vi "Scope Report Event.vi"(8 "error in (no error)":errorcluster, 9 "Event Data":variant, 10 "Scope Events":T1, 11 "I_Scope in":refnum<class "I_Scope.lvclass">) -> (0 "error out":errorcluster, 3 "I_Scope out":refnum<class "I_Scope.lvclass">)   [LabVIEW 2020, in "Actor_Scope.lvlib" / "I_Scope.lvclass"]
uses:
  I_Scope.lvclass
  Actor_Scope/Scope_Event.ctl
  Actor_Scope/Actor_Scope.lvclass
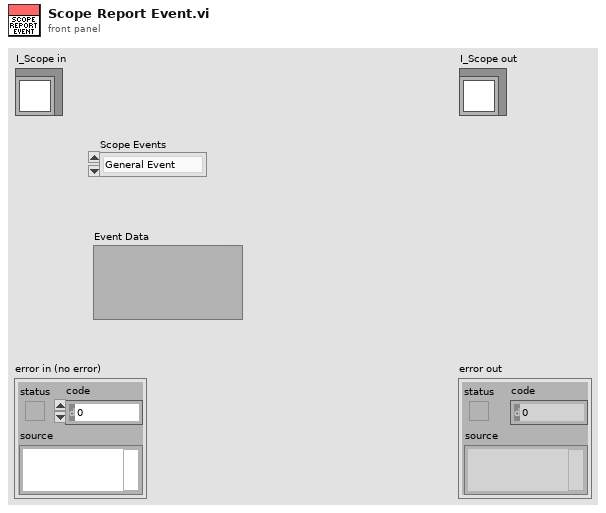
[diagram p1: front panel]
types:
  T1 = typedef "Actor_Scope.lvlib/Actor_Scope.lvclass/Scope_Event.ctl" = enum16{"General Event", "Inited", "Error", "Wfm Acq Complete"}
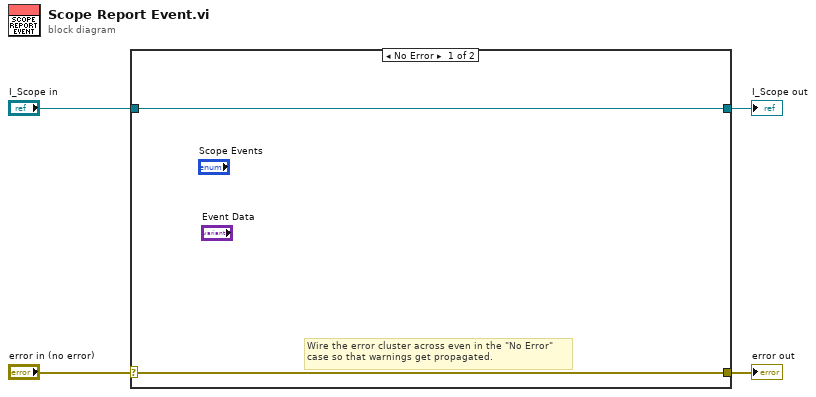
[diagram p0: block diagram]
diagram:
  n1 = case shown="No Error" "error in (no error)" {
    selector: "error in (no error)" -> [w5 w8]
    tunnel: [w5 w8] -> w3
    tunnel: [w6 w7] -> w1
    tunnel: "I_Scope in" -> [w6 w7]
    frame No Error {
      # "Wire the error cluster across even in the \"No Error\"\ncase so that warnings get propagated."
    }
    frame Error {
    }
  }
  "error out" <- w3
  "I_Scope out" <- w1
